vi "ProductDataBase.vi"() -> ()   [LabVIEW 2020]
uses:
  #typedef_Product.ctl
  #typedef_SM_states.ctl
  #typedef_Program_data.ctl
  <vilib>/Utility/file.llb/Write Delimited Spreadsheet (string).vi
panel:
  in  "Open":bool
  in  "What?":string
  in  "Sort":bool
  in  "Search Product":bool
  in  "Next Product":bool
  in  "Remove Product":bool
  in  "Add Product":bool
  in  "Save As":bool
  in  "Stop Program":bool
  in  "Previous Product":bool
  in  "Sort by":enum16{"Number", "Name", "Producer"}(ring)
  in  "Search by":enum16{"Number", "Name", "Producer"}(ring)
  out "Product":T1
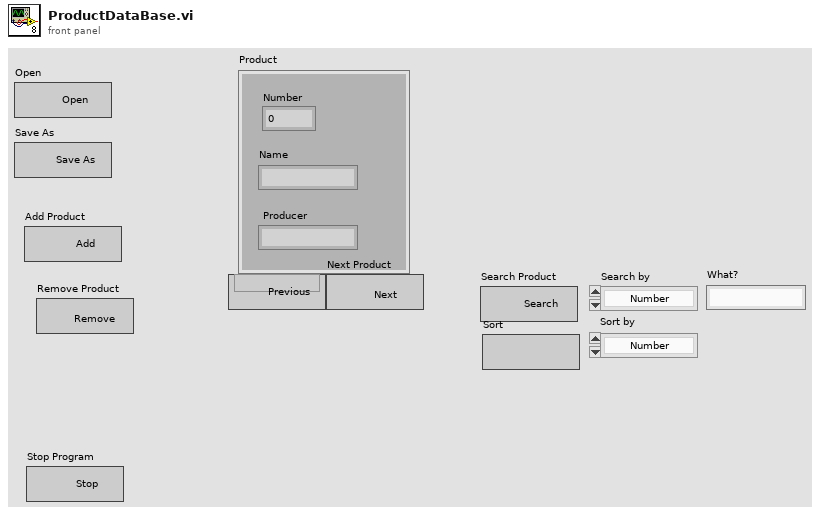
[diagram p1: front panel]
types:
  T1 = typedef "#typedef_Product.ctl" = cluster{"Number":i32, "Name":string, "Producer":string}
  T2 = typedef "#typedef_SM_states.ctl" = enum16{"Initialize", "Idle", "Open", "Previous", "Next", "Save", "Sort", "Search", "Add", "Remove", "Refresh", "Error handler", "Exit"}
  T3 = typedef "#typedef_Program_data.ctl" = cluster{"Products":T1[], "Current Product":i32, "ProductPath":path}
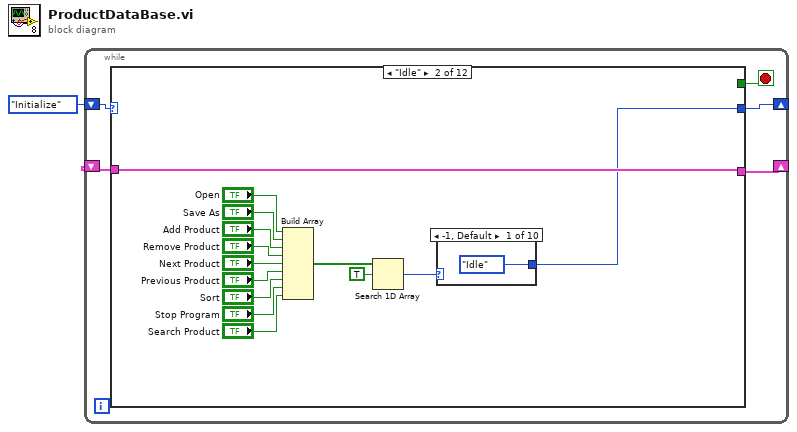
[diagram p0: block diagram]
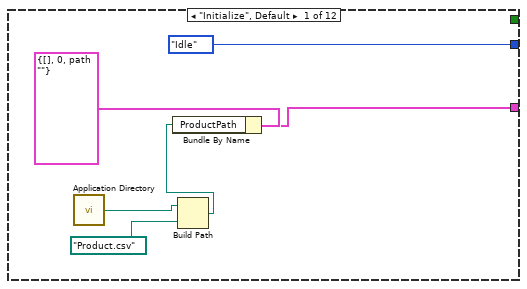
[diagram p2: hidden frame]
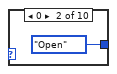
[diagram p3: hidden frame]
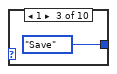
[diagram p4: hidden frame]
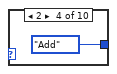
[diagram p5: hidden frame]
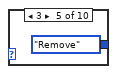
[diagram p6: hidden frame]
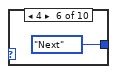
[diagram p7: hidden frame]
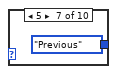
[diagram p8: hidden frame]
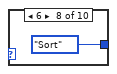
[diagram p9: hidden frame]
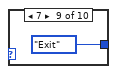
[diagram p10: hidden frame]
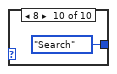
[diagram p11: hidden frame]
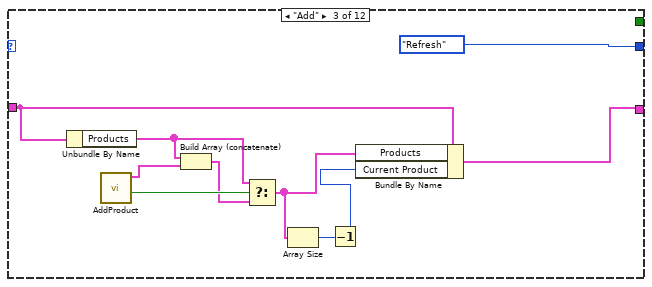
[diagram p12: hidden frame]
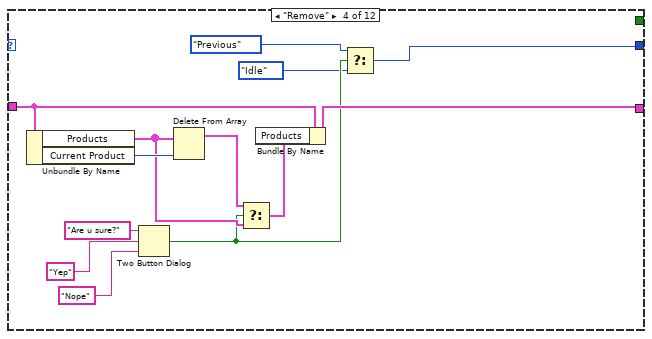
[diagram p13: hidden frame]
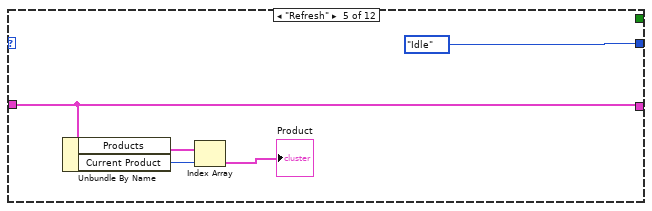
[diagram p14: hidden frame]
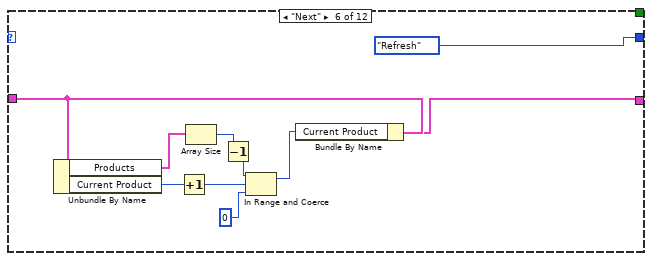
[diagram p15: hidden frame]
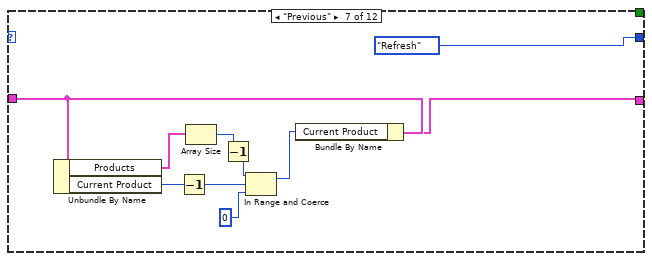
[diagram p16: hidden frame]
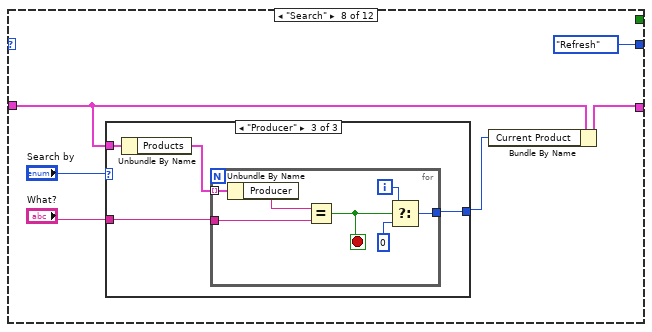
[diagram p17: hidden frame]
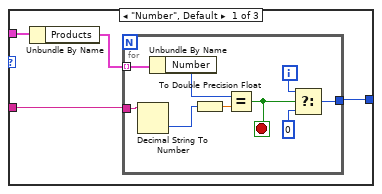
[diagram p18: hidden frame]
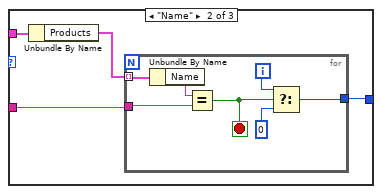
[diagram p19: hidden frame]
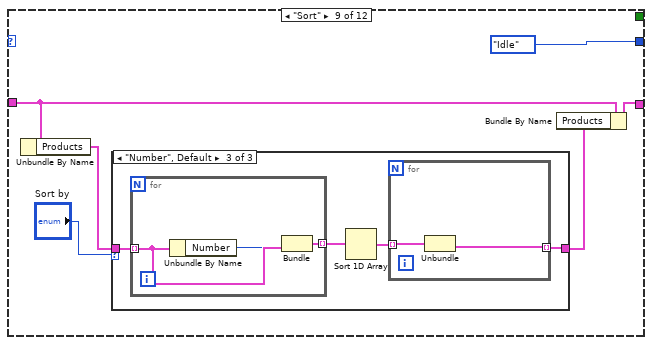
[diagram p20: hidden frame]
diagram:
  n1 = while {
    shift-right: [w4] -> _
    shift-left: #typedef_SM_states."Initialize" ("SM_states") -> [w6]
    shift-right: [w2] -> _
    shift-left: _ -> [w3]
    stop <- w5 stop-if-true
    n2 = case shown="\"Idle\"" w6 {
      tunnel: [_ _ _ _ _ _ _ _ _ _ _ TRUE] -> w5
      tunnel: [#typedef_SM_states."Idle" ("SM_states") w14 #typedef_SM_states."Refresh" ("SM_states") w47 #typedef_SM_states."Idle" ("SM_states") #typedef_SM_states."Refresh" ("SM_states") #typedef_SM_states."Refresh" ("SM_states") #typedef_SM_states."Refresh" ("SM_states") #typedef_SM_states."Idle" ("SM_states") #typedef_SM_states."Idle" ("SM_states") #typedef_SM_states."Idle" ("SM_states") #typedef_SM_states."Exit" ("SM_states")] -> w4
      tunnel: w3 -> [_ w26 w46 w59 w64 w73 w83 w89 w129 w169 w190 w191]
      tunnel: [w10 w26 w41 w57 w64 w66 w76 w87 w128 w169 w186 w191] -> w2
      frame "Initialize", Default {
        n3 = call <vilib>:"Application Directory.vi"() -> ("Application Directory"=w9:path)
        n4 = Build Path(base path=w9, name or relative path=path "Product.csv") -> (appended path=w7:path)
        n5 = Bundle By Name(cluster=T3 {"Products"=[], "Current Product"=0, "ProductPath"=path ""} ("Program Data"), "ProductPath"=w7) -> (w10:T3)
      }
      frame "Idle" {
        n6 = Build Array("Open", "Save As", "Add Product", "Remove Product", "Next Product", "Previous Product", "Sort", "Stop Program", "Search Product") -> (w17:bool[])
        n7 = Search 1D Array(1D array=w17, element=TRUE) -> (index of element=w15:i32)  [unwired: 1 in]
        n8 = case shown="-1, Default" w15 {
          tunnel: [#typedef_SM_states."Idle" ("SM_states") #typedef_SM_states."Open" ("SM_states") #typedef_SM_states."Save" ("SM_states") #typedef_SM_states."Add" ("SM_states") #typedef_SM_states."Remove" ("SM_states") #typedef_SM_states."Next" ("SM_states") #typedef_SM_states."Previous" ("SM_states") #typedef_SM_states."Sort" ("SM_states") #typedef_SM_states."Exit" ("SM_states") #typedef_SM_states."Search" ("SM_states")] -> w14
          frame -1, Default {
          }
          frame 0 {
          }
          frame 1 {
          }
          frame 2 {
          }
          frame 3 {
          }
          frame 4 {
          }
          frame 5 {
          }
          frame 6 {
          }
          frame 7 {
          }
          frame 8 {
          }
        }
      }
      frame "Add" {
        n9 = Unbundle By Name(w46) -> ("Products"=w43:T1[])
        n10 = call "AddProduct.vi"() -> ("Cancelled?"=w44:bool, "New Product"=w45:T1)  [unwired: 8 in, 1 out]
        n11 = Build Array (concatenate)(w43, w45) -> (w42:T1[])
        n12 = Select(t=w43, s=w44, f=w42) -> (s? t:f=w39:T1[])
        n13 = Array Size(array=w39) -> (size(s)=w38:i32)
        n14 = Decrement(x=w38) -> (x-1=w37:i32)
        n15 = Bundle By Name(cluster=w46, "Products"=w39, "Current Product"=w37) -> (w41:T3)
      }
      frame "Remove" {
        n16 = Unbundle By Name(w59) -> ("Products"=w51:T1[], "Current Product"=w58:i32)
        n17 = Two Button Dialog(message="Are u sure?", 1:"Nope" ("F button name (\"Cancel\")"), 2:"Yep" ("F button name (\"Cancel\")")) -> (T button?=w49:bool)
        n18 = Delete From Array(array=w51, index=w58) -> (array with subset deleted=w53:T1[])  [unwired: 1 in, 1 out]
        n19 = Select(t=w53, s=w49, f=w51) -> (s? t:f=w52:T1[])
        n20 = Bundle By Name(cluster=w59, "Products"=w52) -> (w57:T3)
        n21 = Select(t=#typedef_SM_states."Previous" ("SM_states"), s=w49, f=#typedef_SM_states."Idle" ("SM_states")) -> (s? t:f=w47:T2)
      }
      frame "Refresh" {
        n22 = Unbundle By Name(w64) -> ("Products"=w63:T1[], "Current Product"=w60:i32)
        n23 = Index Array(array=w63, index=w60) -> (element=→"Product":T1)
      }
      frame "Next" {
        n24 = Unbundle By Name(w73) -> ("Products"=w69:T1[], "Current Product"=w72:i32)
        n25 = Increment(x=w72) -> (x+1=w71:i32)
        n26 = Array Size(array=w69) -> (size(s)=w68:i32)
        n27 = Decrement(x=w68) -> (x-1=w67:i32)
        n28 = In Range and Coerce(upper limit=w67, x=w71, lower limit=0) -> (coerced(x)=w65:i32)  [unwired: 1 out]
        n29 = Bundle By Name(cluster=w73, "Current Product"=w65) -> (w66:T3)
      }
      frame "Previous" {
        n30 = Unbundle By Name(w83) -> ("Products"=w79:T1[], "Current Product"=w82:i32)
        n31 = Decrement(x=w82) -> (x-1=w81:i32)
        n32 = Array Size(array=w79) -> (size(s)=w78:i32)
        n33 = Decrement(x=w78) -> (x-1=w77:i32)
        n34 = In Range and Coerce(upper limit=w77, x=w81, lower limit=0) -> (coerced(x)=w75:i32)  [unwired: 1 out]
        n35 = Bundle By Name(cluster=w83, "Current Product"=w75) -> (w76:T3)
      }
      frame "Search" {
        n36 = case shown="\"Producer\"" "Search by" {
          tunnel: w89 -> [w94 w107 w118]
          tunnel: "What?" -> [w92 w105 w116]
          tunnel: [w91 w104 w115] -> w86
          frame "Number", Default {
            n37 = Unbundle By Name(w94) -> ("Products"=w93:T1[])
            n38 = for {
              tunnel: w93 -> [w103] mode=indexing
              tunnel: w92 -> [w102]
              tunnel: [w98] -> w91
              i -> [w99]
              stop <- w97 stop-if-true
              n39 = Decimal String To Number(string=w102) -> (number=w101:i32)  [unwired: 2 in, 1 out]
              n40 = Unbundle By Name(w103) -> ("Number"=w100:i32)
              n41 = To Double Precision Float(number=w101) -> (double precision float=w95:dbl)
              n42 = Equal?(x=w100, y=w95) -> (x = y?=w97:bool)
              n43 = Select(t=w99, s=w97, f=0) -> (s? t:f=w98:i32)
            }
          }
          frame "Name" {
            n44 = Unbundle By Name(w107) -> ("Products"=w106:T1[])
            n45 = for {
              tunnel: w106 -> [w114] mode=indexing
              tunnel: w105 -> [w108]
              tunnel: [w111] -> w104
              i -> [w112]
              stop <- w110 stop-if-true
              n46 = Unbundle By Name(w114) -> ("Name"=w113:string)
              n47 = Equal?(x=w113, y=w108) -> (x = y?=w110:bool)
              n48 = Select(t=w112, s=w110, f=0) -> (s? t:f=w111:i32)
            }
          }
          frame "Producer" {
            n49 = Unbundle By Name(w118) -> ("Products"=w117:T1[])
            n50 = for {
              tunnel: w117 -> [w125] mode=indexing
              tunnel: w116 -> [w119]
              tunnel: [w122] -> w115
              i -> [w123]
              stop <- w121 stop-if-true
              n51 = Unbundle By Name(w125) -> ("Producer"=w124:string)
              n52 = Equal?(x=w124, y=w119) -> (x = y?=w121:bool)
              n53 = Select(t=w123, s=w121, f=0) -> (s? t:f=w122:i32)
            }
          }
        }
        n54 = Bundle By Name(cluster=w89, "Current Product"=w86) -> (w87:T3)
      }
      frame "Sort" {
        n55 = Unbundle By Name(w129) -> ("Products"=w131:T1[])
        n56 = case shown="\"Number\", Default" "Sort by" {
          tunnel: w131 -> [w135 w144 w153]
          tunnel: [w132 w141 w150] -> w126
          frame "Name" {
            n57 = for {
              tunnel: w135 -> [w140] mode=indexing
              tunnel: [w138] -> w134 mode=indexing
              n58 = Unbundle By Name(w140) -> ("Name"=w139:string)
              n59 = Bundle("Name"=w139, "Product"=w140) -> (w138:cluster{"Name":string, "Product":T1})  [unwired: 1 in]
            }
            n60 = Sort 1D Array(array=w134) -> (sorted array=w133:cluster{"Name":string, "Product":T1}[])
            n61 = for {
              tunnel: w133 -> [w137] mode=indexing
              tunnel: [w136] -> w132 mode=indexing
              n62 = Unbundle(w137) -> ("Product"=w136:T1)  [unwired: 1 out]
            }
          }
          frame "Producer" {
            n63 = for {
              tunnel: w144 -> [w149] mode=indexing
              tunnel: [w147] -> w143 mode=indexing
              n64 = Unbundle By Name(w149) -> ("Name"=w148:string)
              n65 = Bundle("Name"=w148, "Product"=w149) -> (w147:cluster{"Name":string, "Product":T1})  [unwired: 1 in]
            }
            n66 = Sort 1D Array(array=w143) -> (sorted array=w142:cluster{"Name":string, "Product":T1}[])
            n67 = for {
              tunnel: w142 -> [w146] mode=indexing
              tunnel: [w145] -> w141 mode=indexing
              n68 = Unbundle(w146) -> ("Product"=w145:T1)  [unwired: 1 out]
            }
          }
          frame "Number", Default {
            n69 = for {
              tunnel: w153 -> [w158] mode=indexing
              tunnel: [w156] -> w152 mode=indexing
              n70 = Unbundle By Name(w158) -> ("Number"=w157:i32)
              n71 = Bundle("Number"=w157, "Product"=w158) -> (w156:cluster{"Number":i32, "Product":T1})  [unwired: 1 in]
            }
            n72 = Sort 1D Array(array=w152) -> (sorted array=w151:cluster{"Number":i32, "Product":T1}[])
            n73 = for {
              tunnel: w151 -> [w155] mode=indexing
              tunnel: [w154] -> w150 mode=indexing
              n74 = Unbundle(w155) -> ("Product"=w154:T1)  [unwired: 1 out]
            }
          }
        }
        n75 = Bundle By Name(cluster=w129, "Products"=w126) -> (w128:T3)
      }
      frame "Save" {
        n76 = Unbundle By Name(w169) -> ("Products"=w167:T1[], "ProductPath"=w164:path)
        n77 = Build Array("NumerProduktu", "NazwaProduktu", "Producent") -> (w160:string[])
        n78 = call-poly <vilib>:"Write Delimited Spreadsheet.vi"("file path (dialog if empty)"=w164, "1D data"=w160, "append to file? (new file:F)"=TRUE, "delimiter (\\t)"="," ("delimiter (\\t)")) -> ("new file path (Not A Path if cancelled)"=w159:path)  [unwired: 10 in, 1 out]
        n79 = for {
          tunnel: w167 -> [w184] mode=indexing
          tunnel: w167 -> [w182]
          shift-right: [w171] -> _
          shift-left: w159 -> [w175]
          i -> [w180]
          stop <- w178 stop-if-true
          n80 = Array Size(array=w182) -> (size(s)=w181:i32)
          n81 = Unbundle By Name(w184) -> ("Number"=w183:i32, "Name"=w177:string, "Producer"=w176:string)
          n82 = Decrement(x=w181) -> (x-1=w179:i32)
          n83 = Equal?(x=w179, y=w180) -> (x = y?=w178:bool)
          n84 = Number To Decimal String(number=w183) -> (decimal integer string=w170:string)  [unwired: 1 in]
          n85 = Build Array(w170, w177, w176) -> (w174:string[])
          n86 = call-poly <vilib>:"Write Delimited Spreadsheet.vi"("file path (dialog if empty)"=w175, "1D data"=w174, "append to file? (new file:F)"=TRUE, "delimiter (\\t)"="," ("delimiter (\\t)")) -> ("new file path (Not A Path if cancelled)"=w171:path)  [unwired: 10 in, 1 out]
        }
      }
      frame "Open" {
        n87 = Unbundle By Name(w190) -> ("Products"=w187:T1[], "ProductPath"=w188:path)
        n88 = Read from Binary File(5:w187, 11:w188) -> (2:w185:T1[])  [unwired: 4 in, 3 out]
        n89 = Bundle By Name(cluster=w190, "Products"=w185) -> (w186:T3)
      }
      frame "Exit" {
      }
    }
  }
